vi "getGratingPosition.vi"(6 "Delay between send and receive [ms]":i32=100, 8 "error in (no error)":errorcluster, 11 "Monochromator in":refnum<class "Monochromator.lvclass">) -> (0 "error out":errorcluster, 2 "position":i32, 3 "Monochromator out":refnum<class "Monochromator.lvclass">)   [LabVIEW 2023, in "Monochromator.lvclass"]
uses:
  Monochromator.lvclass
  d9b87029-586e-44ee-a6e5-d4a5e0edce38.vi
  b59fd1e7-dcda-425c-bd6c-61aafb79e7f4.vi
  GenericDevice/GenericDevice.lvclass
  <vilib>/IlluminatedG/lv-web-crypto/lv-json/JSON/JSON.lvlib
  GratingPosition.ctl
panel:
  # "Connector Pane"
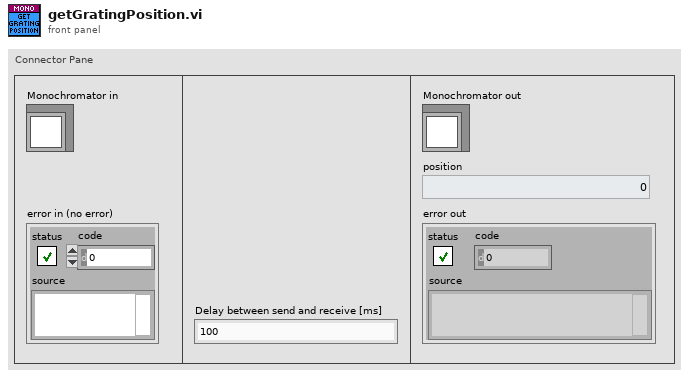
[diagram p1: front panel]
types:
  T1 = typedef "Monochromator.lvclass/GratingPosition.ctl" = cluster{"position":i32}
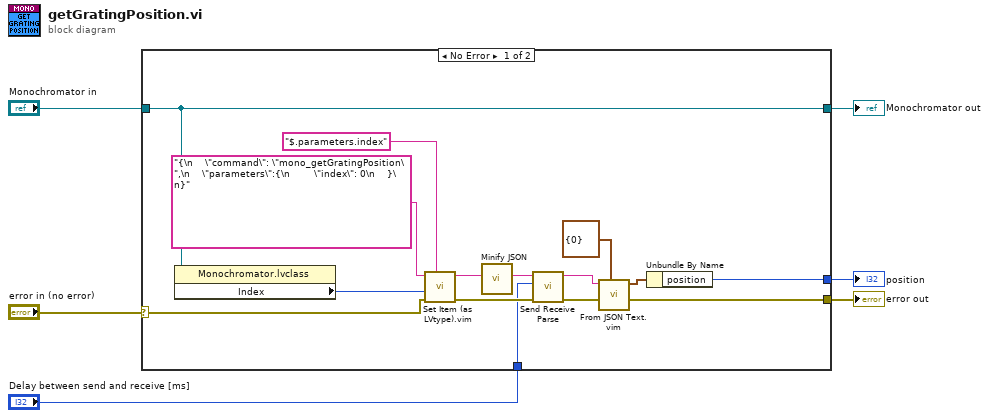
[diagram p0: block diagram]
diagram:
  n1 = case shown="No Error" "error in (no error)" {
    selector: "error in (no error)" -> [w17 w23]
    tunnel: [w16 w23] -> w5
    tunnel: [w19 w22] -> w3
    tunnel: "Monochromator in" -> [w19 w22]
    tunnel: [w9 _] -> w2
    tunnel: "Delay between send and receive [ms]" -> [w7 _]
    frame No Error {
      n2 = property class="Monochromator.lvclass"(reference=w19) -> ("Index"=w18:i32)  [unwired: 1 in, 2 out]
      n3 = call "Set Item (as LVtype).vim"("$Path or Item Name"="$.parameters.index", "error in (no error)"=w17, "Anything"=w18, "JSON"="{\n    \"command\": \"mono_getGratingPosition\",\n    \"parameters\":{\n        \"index\": 0\n    }\n}") -> ("error out"=w15:errorcluster, "<JSON>"=w12:string)  [unwired: 4 in, 1 out]
      n4 = call <vilib>:"Minify JSON.vi"("JSON String"=w12) -> ("Minified JSON"=w11:string)  [unwired: 10 in]
      n5 = call "Send Receive Parse.vi"("error in"=w15, "Delay between send and receive [ms]"=w7, "<JSON>"=w11) -> ("error out"=w13:errorcluster, "results-JSON string"=w14:string)  [unwired: 6 in, 1 out]
      n6 = call "From JSON Text.vim"("Data Type and Default Value"=T1 {"position"=0} ("Grating Position"), "error in (no error)"=w13, "JSON"=w14) -> ("error out"=w16:errorcluster, "Data out"=w10:T1)  [unwired: 7 in]
      n7 = Unbundle By Name(w10) -> ("position"=w9:i32)
    }
    frame Error {
    }
  }
  "error out" <- w5
  "Monochromator out" <- w3
  "position" <- w2
